vi "Untitled 1.vi"() -> ()   [LabVIEW 2017]
panel:
  out "Array":i32[](array[numeric])
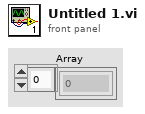
[diagram p1: front panel]
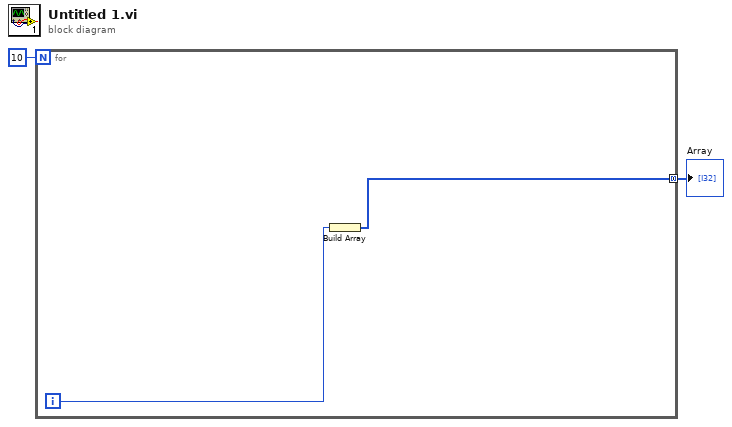
[diagram p0: block diagram]
diagram:
  n1 = for {
    N: 10 -> [_]
    tunnel: [w4] -> w1 mode=concatenating
    i -> [w3]
    n2 = Build Array(w3) -> (w4:i32[])
  }
  "Array" <- w1
